vi "Notification user LV2.vi"(0 "Data":T1, 11 "Error In":errorcluster, 13 "Operation":T2) -> (4 "Message type":refnum<user-event>, 15 "Error Out":errorcluster)   [LabVIEW 2020]
doc: "User LV2 to propagate the notification reference."
uses:
  Transmitter/Typedefs/User_Event_Operation.ctl
  Transmitter/Typedefs/Message type data.ctl
  Transmitter/Data Communication Transmitter.lvlib
panel:
  # "Message Type User Event"
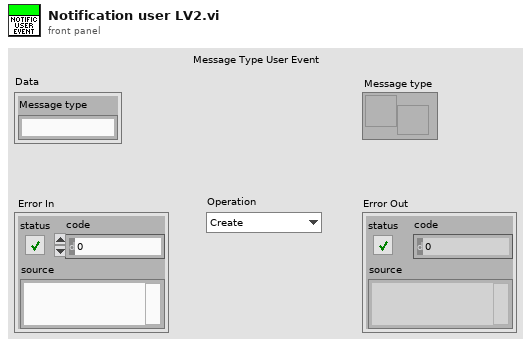
[diagram p1: front panel]
types:
  T1 = typedef "Data Communication Transmitter.lvlib/Message type data.ctl" = cluster{"Message type":string}
  T2 = typedef "Data Communication Transmitter.lvlib/User_Event_Operation.ctl" = enum16{"Create", "Generate", "Destroy", "Get Ref"}
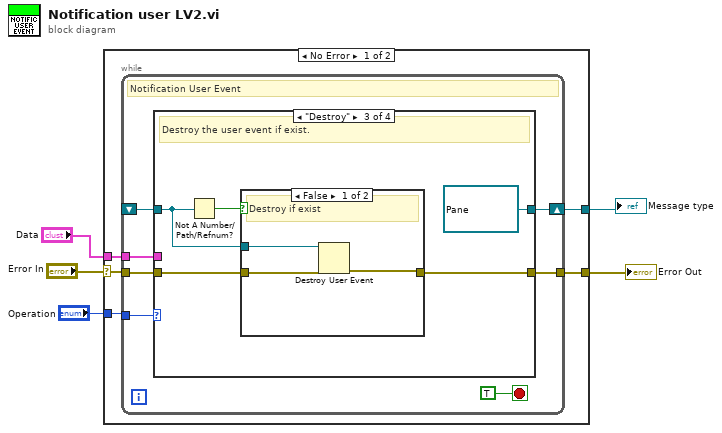
[diagram p0: block diagram]
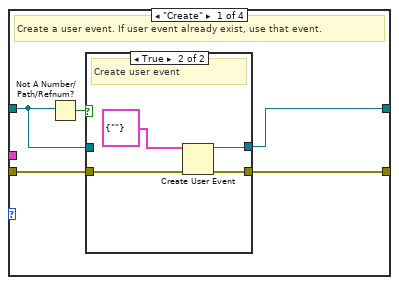
[diagram p2: hidden frame]
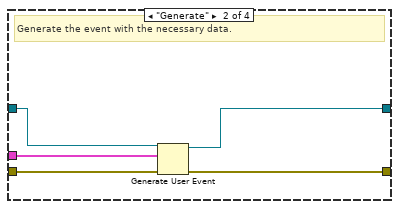
[diagram p4: hidden frame]
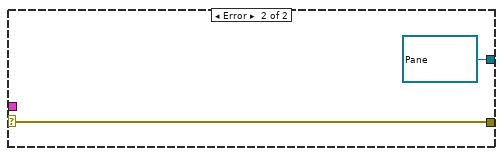
[diagram p7: hidden frame]
diagram:
  n1 = case shown="No Error" "Error In" {
    selector: "Error In" -> [w8 w46]
    tunnel: "Operation" -> [w10 _]
    tunnel: [w9 w46] -> w4
    tunnel: "Data" -> [w7 _]
    tunnel: [w6 refnum<user-event> refnum ("Data")] -> w1
    frame No Error {
      n2 = while {
        tunnel: w10 -> [w17]
        shift-right: [w16] -> w6
        shift-left: _ -> [w15]
        tunnel: w8 -> [w14]
        tunnel: [w13] -> w9
        tunnel: w7 -> [w11]
        stop <- TRUE stop-if-true
        # "Notification User Event"
        n3 = case shown="\"Destroy\"" w17 {
          tunnel: [w18 w30 refnum<user-event> refnum ("Data") w44] -> w16
          tunnel: w15 -> [w19 w31 w35 w44]
          tunnel: w14 -> [w21 w33 w37 w43]
          tunnel: [w20 w32 w36 w43] -> w13
          tunnel: w11 -> [_ w29 _ _]
          frame "Create" {
            # "Create a user event. If user event already exist, use that event."
            n4 = Not A Number/Path/Refnum?(number/path/refnum=w19) -> (NaN/Path/Refnum?=w22:bool)
            n5 = case shown="True" w22 {
              tunnel: [w24 w28] -> w18
              tunnel: w21 -> [w23 w27]
              tunnel: [w23 w26] -> w20
              tunnel: w19 -> [w24 _]
              frame False {
                # "Already exist"
              }
              frame True {
                # "Create user event"
                n6 = Create User Event(user event datatype=T1 {"Message type"=""} ("Data"), error in=w27) -> (user event=w28:refnum<user-event>, error out=w26:errorcluster)
              }
            }
          }
          frame "Generate" {
            # "Generate the event with the necessary data."
            n7 = Generate User Event(user event=w31, event data cluster=w29, error in=w33) -> (user event out=w30:refnum<user-event>, error out=w32:errorcluster)  [unwired: 1 in]
          }
          frame "Destroy" {
            # "Destroy the user event if exist."
            n8 = Not A Number/Path/Refnum?(number/path/refnum=w35) -> (NaN/Path/Refnum?=w38:bool)
            n9 = case shown="False" w38 {
              tunnel: w37 -> [w41 w42]
              tunnel: [w40 w42] -> w36
              tunnel: w35 -> [w39 _]
              frame False {
                # "Destroy if exist"
                n10 = Destroy User Event(user event=w39, error in=w41) -> (error out=w40:errorcluster)
              }
              frame True {
                # "User Event doesnot exist"
              }
            }
          }
          frame "Get Ref" {
            # "Get the User Event Reference"
          }
        }
      }
    }
    frame Error {
    }
  }
  "Error Out" <- w4
  "Message type" <- w1
